vi "Plot 2 testing.vi"(8 "error in":errorcluster, 10 "TWT type":string="PT6109 Input", 11 "XY Graph":refnum<vi>) -> (0 "error out":errorcluster, 2 "concatenated string 6":string, 3 "Plot 2 pass?":bool)   [LabVIEW 2014]
panel:
  out "Plot 2 pass?":T1
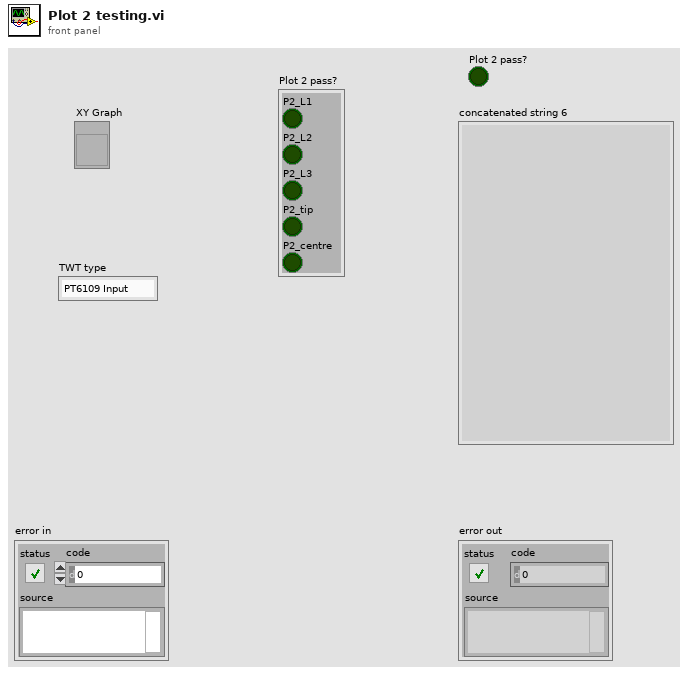
[diagram p1: front panel]
types:
  T1 = cluster{"P2_L1":bool, "P2_L2":bool, "P2_L3":bool, "P2_tip":bool, "P2_centre":bool}
  T2 = enum16{"get TWT types", "read TWT spec.", "save TWT spec.", "remove TWT spec."}
  T3 = typedef "TWT spec..ctl" = cluster{"Reference level":dbl, "L1 min":dbl, "L1 max":dbl, "L2 min":dbl, "L2 max":dbl, "L3 min":dbl, "L3 max":dbl, "Tip loss nominal":dbl, "Tip loss min":dbl, "Tip loss max":dbl, "Centre loss nominal":dbl, "Centre loss min":dbl, "Centre loss max":dbl}
  T4 = typedef "dist. between cursors.ctl" = cluster{"0 to c1":dbl, "c1 to c2":dbl, "c1 to c3":dbl, "c3 to c4":dbl}
  T5 = cluster{"Plot 1 distances":T4, "Plot 2 distances":T4, "Plot 3 distances":T4}
  T6 = typedef "LVAnnotationListTypeDef.ctl" = cluster{"Name":string, "Color":u32, "Style":u8, "Point Style":u8, "Name Visible":bool, "Allow Drag":bool, "Annotation Mode":u32, "Plot":i32, "Index":i32, "Position":cluster{"X":dbl, "Y":dbl}, "X Scale":u32, "Y Scale":u32, "Show Arrow":bool, "Lock Name":bool, "Plot Area":i32, "Label Offset":cluster{"X":dbl, "Y":dbl}}[]
  T7 = cluster{"Name":string, "Color":u32, "Style":u8, "Point Style":u8, "Name Visible":bool, "Allow Drag":bool, "Annotation Mode":u32, "Plot":i32, "Index":i32, "Position":cluster{"X":dbl, "Y":dbl}, "X Scale":u32, "Y Scale":u32, "Show Arrow":bool, "Lock Name":bool, "Plot Area":i32, "Label Offset":cluster{"X":dbl, "Y":dbl}}
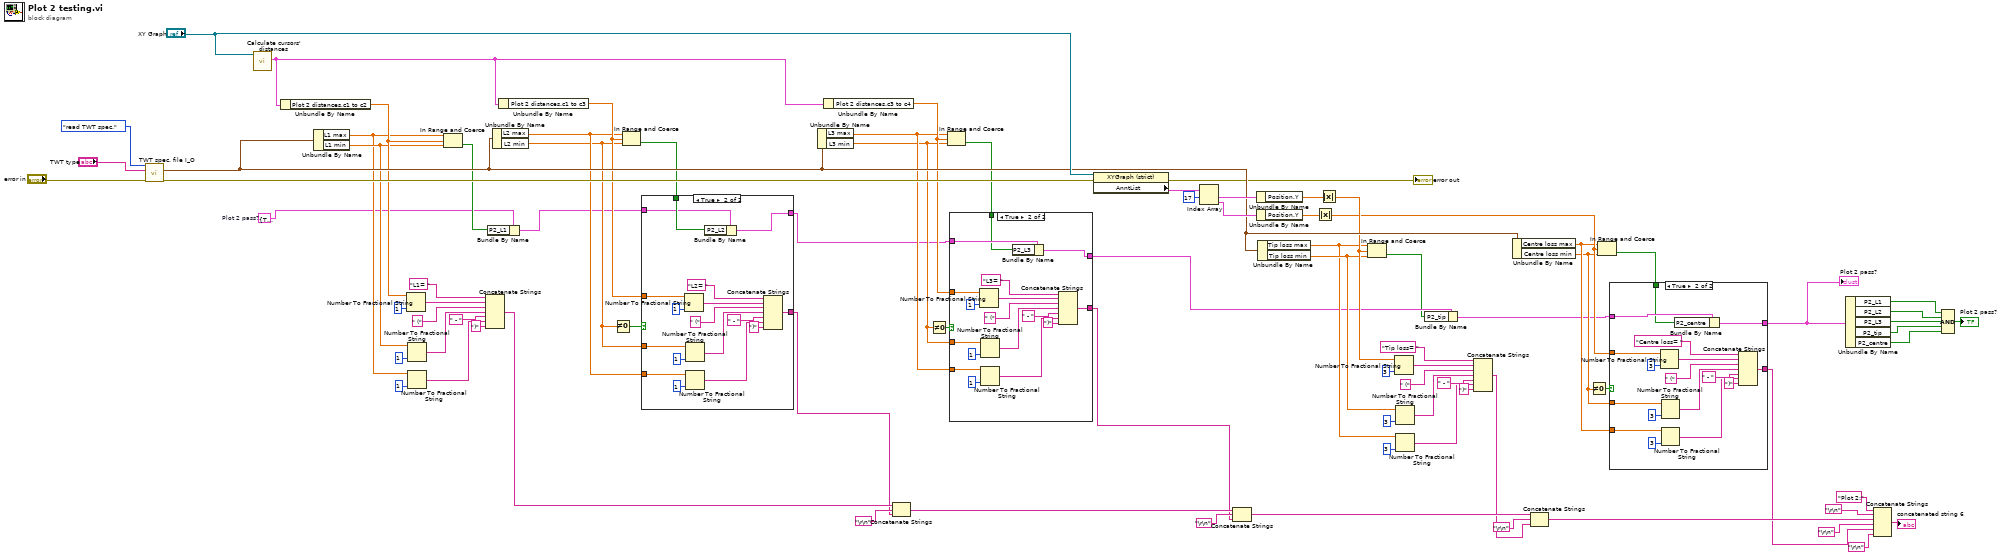
[diagram p0: block diagram]
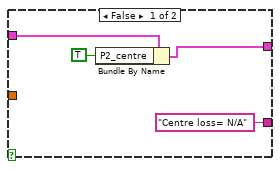
[diagram p2: hidden frame]
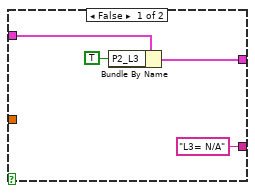
[diagram p3: hidden frame]
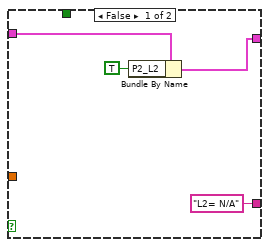
[diagram p4: hidden frame]
diagram:
  w15 = T1 {"P2_L1"=TRUE, "P2_L2"=TRUE, "P2_L3"=TRUE, "P2_tip"=TRUE, "P2_centre"=TRUE}  # Plot 2 pass?
  n1 = call "TWT spec. file I_O.vi"("error in"="error in", "TWT type"="TWT type", "Enum"=T2."read TWT spec.") -> ("error out"=w81:errorcluster, "TWT spec"=w74:T3)  [unwired: 6 in, 1 out]
  n2 = call "Calculate cursors' distances.vi"("XY Graph"="XY Graph") -> ("All cursors' dist."=w82:T5)  [unwired: 9 in, 1 out]
  n3 = Unbundle By Name(w82) -> ("Plot 2 distances.c1 to c2"=w68:dbl)
  n4 = Unbundle By Name(w74) -> ("L1 max"=w64:dbl, "L1 min"=w65:dbl)
  n5 = Number To Fractional String(number=w68, precision (6)=i16 1) -> (F-format string=w70:string)  [unwired: 2 in]
  n6 = Number To Fractional String(number=w65, precision (6)=i16 1) -> (F-format string=w62:string)  [unwired: 2 in]
  n7 = Number To Fractional String(number=w64, precision (6)=i16 1) -> (F-format string=w60:string)  [unwired: 2 in]
  n8 = In Range and Coerce(upper limit=w64, x=w68, lower limit=w65) -> (In Range?=w17:bool)  [unwired: 1 out]
  n9 = Concatenate Strings("L1= " ("string"), w70, " (" ("string"), w62, " - " ("string"), w60, ")" ("string")) -> (w33:string)
  n10 = Bundle By Name(cluster=w15, "P2_L1"=w17) -> (w14:T1)
  n11 = Unbundle By Name(w74) -> ("L2 max"=w57:dbl, "L2 min"=w38:dbl)
  n12 = Unbundle By Name(w82) -> ("Plot 2 distances.c1 to c3"=w58:dbl)
  n13 = Not Equal To 0?(x=w38) -> (x != 0?=w39:bool)
  n14 = In Range and Coerce(upper limit=w57, x=w58, lower limit=w38) -> (In Range?=w16:bool)  [unwired: 1 out]
  n15 = case shown="True" w39 {
    tunnel: ["L2= N/A" w96] -> w31
    tunnel: w58 -> [_ w95]
    tunnel: w38 -> [_ w94]
    tunnel: w57 -> [_ w93]
    tunnel: w16 -> [_ w92]
    tunnel: w14 -> [w88 w91]
    tunnel: [w86 w90] -> w13
    frame False {
      n16 = Bundle By Name(cluster=w88, "P2_L2"=TRUE) -> (w86:T1)
    }
    frame True {
      n17 = Number To Fractional String(number=w95, precision (6)=i16 1) -> (F-format string=w105:string)  [unwired: 2 in]
      n18 = Number To Fractional String(number=w94, precision (6)=i16 1) -> (F-format string=w100:string)  [unwired: 2 in]
      n19 = Number To Fractional String(number=w93, precision (6)=i16 1) -> (F-format string=w98:string)  [unwired: 2 in]
      n20 = Bundle By Name(cluster=w91, "P2_L2"=w92) -> (w90:T1)
      n21 = Concatenate Strings("L2= " ("string"), w105, " (" ("string"), w100, " - " ("string"), w98, ")" ("string")) -> (w96:string)
    }
  }
  n22 = Unbundle By Name(w74) -> ("L3 max"=w55:dbl, "L3 min"=w36:dbl)
  n23 = Unbundle By Name(w82) -> ("Plot 2 distances.c3 to c4"=w56:dbl)
  n24 = Concatenate Strings(w33, "\r\n", w31) -> (w29:string)
  n25 = Not Equal To 0?(x=w36) -> (x != 0?=w37:bool)
  n26 = In Range and Coerce(upper limit=w55, x=w56, lower limit=w36) -> (In Range?=w12:bool)  [unwired: 1 out]
  n27 = case shown="True" w37 {
    tunnel: ["L3= N/A" w127] -> w28
    tunnel: w56 -> [_ w116]
    tunnel: w36 -> [_ w115]
    tunnel: w55 -> [_ w114]
    tunnel: w13 -> [w108 w113]
    tunnel: [w107 w112] -> w11
    tunnel: w12 -> [_ w111]
    frame False {
      n28 = Bundle By Name(cluster=w108, "P2_L3"=TRUE ("P2_L2")) -> (w107:T1)
    }
    frame True {
      n29 = Number To Fractional String(number=w116, precision (6)=i16 1) -> (F-format string=w118:string)  [unwired: 2 in]
      n30 = Number To Fractional String(number=w115, precision (6)=i16 1) -> (F-format string=w123:string)  [unwired: 2 in]
      n31 = Number To Fractional String(number=w114, precision (6)=i16 1) -> (F-format string=w125:string)  [unwired: 2 in]
      n32 = Bundle By Name(cluster=w113, "P2_L3"=w111) -> (w112:T1)
      n33 = Concatenate Strings("L3= " ("string"), w118, " (" ("string"), w123, " - " ("string"), w125, ")" ("string")) -> (w127:string)
    }
  }
  n34 = property class="XYGraph (strict)"(reference="XY Graph", error in=w81) -> (error out=→"error out":errorcluster, "AnntList"=w79:T6)  [unwired: 1 out]
  n35 = Index Array(array=w79, index #1=17 ("index")) -> (element #1=w77:T7, element #2=w76:T7)  [unwired: 1 in]
  n36 = Concatenate Strings(w29, "\r\n", w28) -> (w26:string)
  n37 = Unbundle By Name(w77) -> ("Position.Y"=w75:dbl)
  n38 = Unbundle By Name(w76) -> ("Position.Y"=w73:dbl)
  n39 = Unbundle By Name(w74) -> ("Tip loss max"=w42:dbl, "Tip loss min"=w43:dbl)
  n40 = Absolute Value(x=w73) -> (abs(x)=w41:dbl)
  n41 = Absolute Value(x=w75) -> (abs(x)=w44:dbl)
  n42 = In Range and Coerce(upper limit=w42, x=w44, lower limit=w43) -> (In Range?=w10:bool)  [unwired: 1 out]
  n43 = Number To Fractional String(number=w44, precision (6)=i16 3) -> (F-format string=w53:string)  [unwired: 2 in]
  n44 = Number To Fractional String(number=w43, precision (6)=i16 3) -> (F-format string=w48:string)  [unwired: 2 in]
  n45 = Number To Fractional String(number=w42, precision (6)=i16 3) -> (F-format string=w46:string)  [unwired: 2 in]
  n46 = Bundle By Name(cluster=w11, "P2_tip"=w10) -> (w9:T1)
  n47 = Concatenate Strings("Tip loss= " ("string"), w53, " (" ("string"), w48, " - " ("string"), w46, ")" ("string")) -> (w25:string)
  n48 = Unbundle By Name(w74) -> ("Centre loss max"=w40:dbl, "Centre loss min"=w34:dbl)
  n49 = Concatenate Strings(w26, "\r\n", w25) -> (w23:string)
  n50 = Not Equal To 0?(x=w34) -> (x != 0?=w35:bool)
  n51 = In Range and Coerce(upper limit=w40, x=w41, lower limit=w34) -> (In Range?=w8:bool)  [unwired: 1 out]
  n52 = case shown="True" w35 {
    tunnel: ["Centre loss= N/A" w138] -> w22
    tunnel: w41 -> [_ w137]
    tunnel: w34 -> [_ w136]
    tunnel: w40 -> [_ w135]
    tunnel: w9 -> [w130 w134]
    tunnel: w8 -> [_ w133]
    tunnel: [w128 w132] -> w1
    frame False {
      n53 = Bundle By Name(cluster=w130, "P2_centre"=TRUE) -> (w128:T1)
    }
    frame True {
      n54 = Number To Fractional String(number=w137, precision (6)=i16 3) -> (F-format string=w147:string)  [unwired: 2 in]
      n55 = Number To Fractional String(number=w136, precision (6)=i16 3) -> (F-format string=w142:string)  [unwired: 2 in]
      n56 = Number To Fractional String(number=w135, precision (6)=i16 3) -> (F-format string=w140:string)  [unwired: 2 in]
      n57 = Bundle By Name(cluster=w134, "P2_centre"=w133) -> (w132:T1)
      n58 = Concatenate Strings("Centre loss= " ("string"), w147, " (" ("string"), w142, " - " ("string"), w140, ")" ("string")) -> (w138:string)
    }
  }
  "Plot 2 pass?" <- w1
  n59 = Unbundle By Name(w1) -> ("P2_L1"=w7:bool, "P2_L2"=w6:bool, "P2_L3"=w5:bool, "P2_tip"=w4:bool, "P2_centre"=w3:bool)
  n60 = Concatenate Strings("Plot 2:" ("string"), "\r\n", w23, "\r\n", w22, "\r\n") -> (→"concatenated string 6":string)
  n61 = Compound Arithmetic op=AND(w7, w6, w5, w4, w3) -> (→"Plot 2 pass?":bool)
